vi "ATF-Pump-RT_DAQ.vi"(8 "error in":errorcluster, 11 "Data FIFO Ref":T1) -> (0 "error out":errorcluster)   [LabVIEW 2022 SP3]
uses:
  RT Controls/ATF-Pump-Data FIFO.ctl
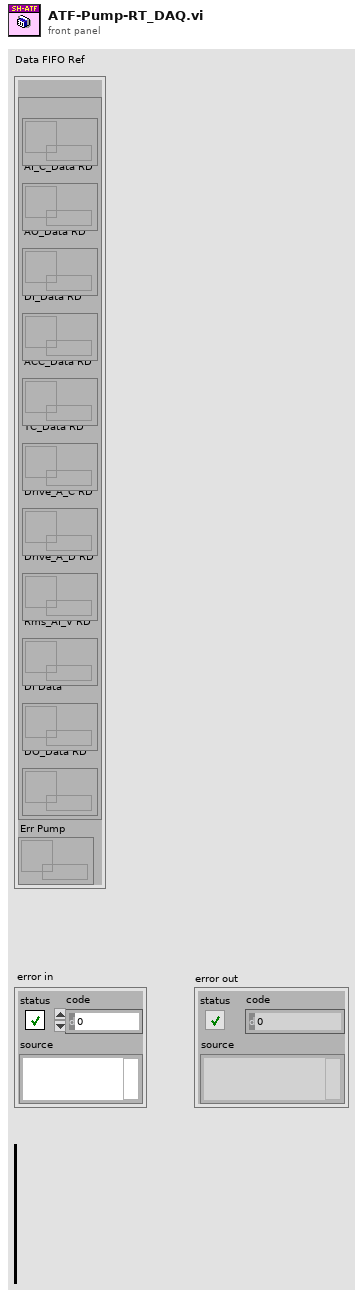
[diagram p1: front panel]
types:
  T1 = typedef "ATF-Pump-Data FIFO.ctl" = cluster{"RD":cluster{"AI_V_Data RD":refnum<queue>, "AI_C_Data RD":refnum<queue>, "AO_Data RD":refnum<queue>, "DI_Data RD":refnum<queue>, "ACC_Data RD":refnum<queue>, "TC_Data RD":refnum<queue>, "Drive_A_C RD":refnum<queue>, "Drive_A_D RD":refnum<queue>, "Rms_AI_V RD":refnum<queue>, "DI Data":refnum<queue>, "DO_Data RD":refnum<queue>}, "Err Pump":refnum<queue>}
  T2 = cluster{"Config":cluster{"AO config":cluster{"Channel_Name":string, "Channel_Number":string, "Default_Value":dbl, "Units":string}[], "AI config":cluster{"Channel_Name":string, "Channel_Number":string, "Pre_Scale_min":dbl, "Pre_Scale_max":dbl, "Sensor_min":dbl, "Sensor_max":dbl, "Units":string}[], "DI config":cluster{"Channel_Name":string, "Channel_Number":string, "Default_Value":bool, "DI invert?":bool}[], "DO config":cluster{"Channel_Name":string, "Channel_Number":string, "Default_Value":bool, "DO invert?":bool}[], "TC config":cluster{"Channel_Name":string, "Channel_Number":string, "Pre_Scale_min":dbl, "Pre_Scale_max":dbl, "units":i32, " type":i32}[], "ACC config":cluster{"Channel_Name":string, "Channel_Number":string, "Pre_Scale_min":dbl, "Pre_Scale_max":dbl, "Terminal configuration":i32, "Sensitivity":dbl, "Sensitivity units":i32}[], "SG config":cluster{"Channel_Name":string, "Channel_Number":string, "Pre_Scale_min":dbl, "Pre_Scale_max":dbl}[], "Strain Gauge Settings":cluster{"poisson ratio":dbl, "nominal gage resistance":dbl, "gage factor":dbl}, "Bridge Settings":cluster{"voltage excitation value":dbl, "voltage excitation source":i32, "initial bridge voltage":dbl, "lead wire resistance":dbl, "strain configuration":i32}, "Sample Rate":cluster{"AI Sample Rate":dbl[], "AO Sample Rate":dbl[], "DI Sample Rate":dbl[], "TC Sample Rate":dbl[], "DO Sample Rate":dbl[], "SG Sample Rate":dbl[], "ACC Sample Rate":dbl[]}}, "FIFO Ref":T1, "AI_Task":refnum<k21>, "AO_Task":refnum<k21>, "DI_Task":refnum<k21>, "DO_Task":refnum<k21>, "ACC_Task":refnum<k21>, "TC_Task":refnum<k21>, "AI_V_Task":refnum<k21>}
  T3 = enum16{"Initialize", "Create Task", "Start", "Acquire", "Stop", "Exit"}
  T4 = cluster{"Start DAQ":bool, "Stop DAQ":bool, "RT Stop":bool, "RT Exit":bool, "Start Seq":bool}
  T5 = cluster{"AO config":cluster{"Channel_Name":string, "Channel_Number":string, "Default_Value":dbl, "Units":string}[], "AI config":cluster{"Channel_Name":string, "Channel_Number":string, "Pre_Scale_min":dbl, "Pre_Scale_max":dbl, "Sensor_min":dbl, "Sensor_max":dbl, "Units":string}[], "DI config":cluster{"Channel_Name":string, "Channel_Number":string, "Default_Value":bool, "DI invert?":bool}[], "DO config":cluster{"Channel_Name":string, "Channel_Number":string, "Default_Value":bool, "DO invert?":bool}[], "TC config":cluster{"Channel_Name":string, "Channel_Number":string, "Pre_Scale_min":dbl, "Pre_Scale_max":dbl, "units":i32, "thermocouple type":i32}[], "ACC config":cluster{"Channel_Name":string, "Channel_Number":string, "Pre_Scale_min":dbl, "Pre_Scale_max":dbl, "Terminal configuration":i32, "Sensitivity":dbl, "Sensitivity units":i32}[], "SG config":cluster{"Channel_Name":string, "Channel_Number":string, "Pre_Scale_min":dbl, "Pre_Scale_max":dbl}[], "Strain Gauge Settings":cluster{"poisson ratio":dbl, "nominal gage resistance":dbl, "gage factor":dbl}, "Bridge Settings":cluster{"voltage excitation value":dbl, "voltage excitation source":i32, "initial bridge voltage":dbl, "lead wire resistance":dbl, "strain configuration":i32}, "Sample Rate":cluster{"AI Sample Rate":dbl[], "AO Sample Rate":dbl[], "DI Sample Rate":dbl[], "TC Sample Rate":dbl[], "DO Sample Rate":dbl[], "SG Sample Rate":dbl[], "ACC Sample Rate":dbl[]}}
  T6 = cluster{"Channel_Name":string, "Channel_Number":string, "Pre_Scale_min":dbl, "Pre_Scale_max":dbl, "Sensor_min":dbl, "Sensor_max":dbl, "Units":string}[]
  T7 = cluster{"Channel_Name":string, "Channel_Number":string, "Default_Value":dbl, "Units":string}[]
  T8 = cluster{"Channel_Name":string, "Channel_Number":string, "Default_Value":bool, "DI invert?":bool}[]
  T9 = cluster{"Channel_Name":string, "Channel_Number":string, "Default_Value":bool, "DO invert?":bool}[]
  T10 = cluster{"Channel_Name":string, "Channel_Number":string, "Pre_Scale_min":dbl, "Pre_Scale_max":dbl, "Terminal configuration":i32, "Sensitivity":dbl, "Sensitivity units":i32}[]
  T11 = cluster{"Channel_Name":string, "Channel_Number":string, "Pre_Scale_min":dbl, "Pre_Scale_max":dbl, "units":i32, " type":i32}[]
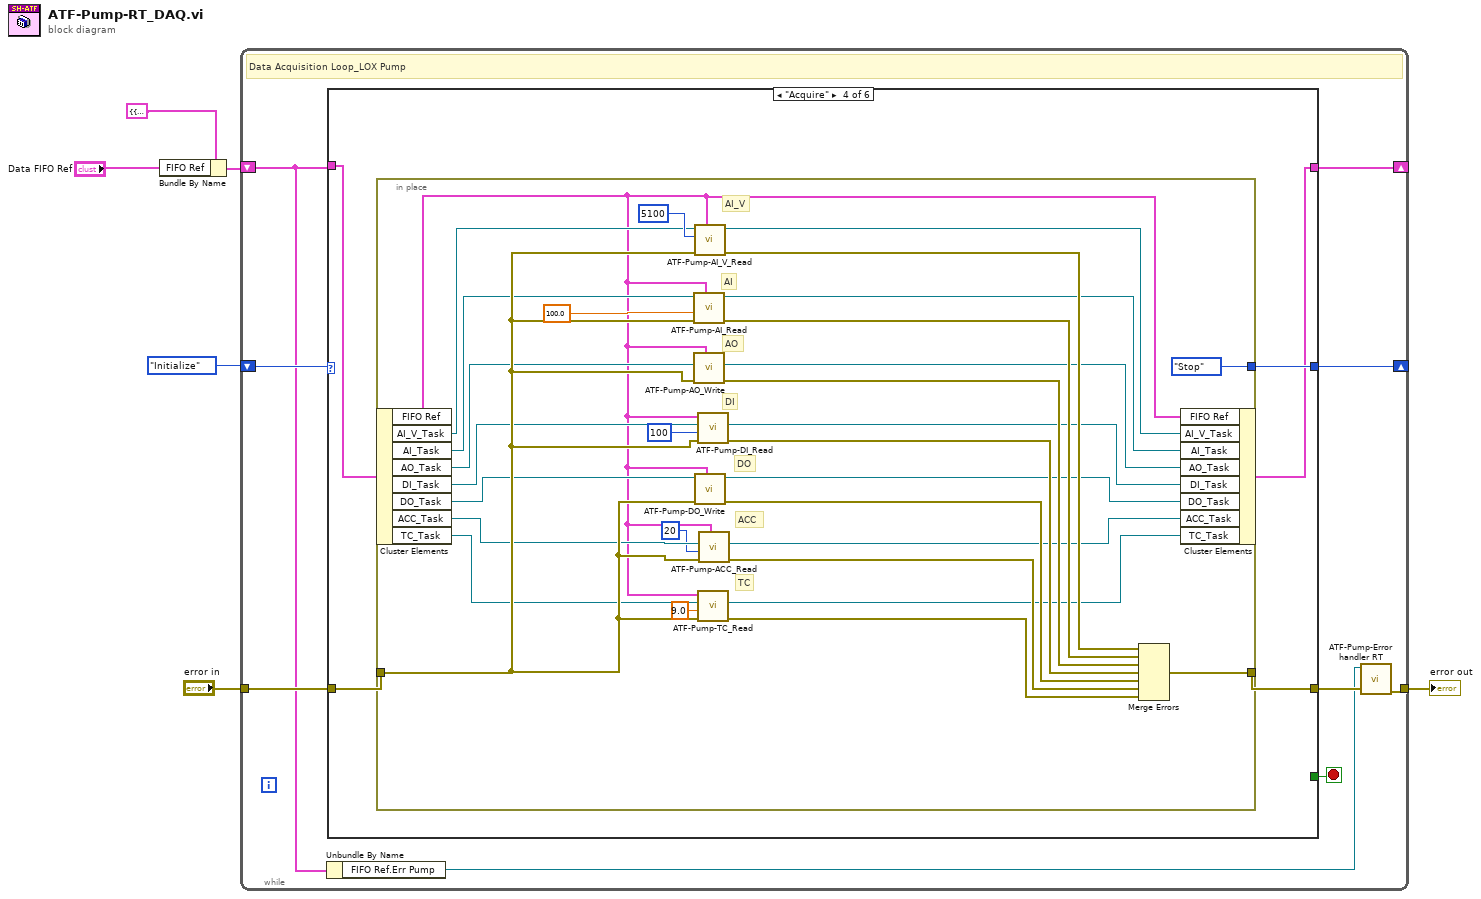
[diagram p0: block diagram]
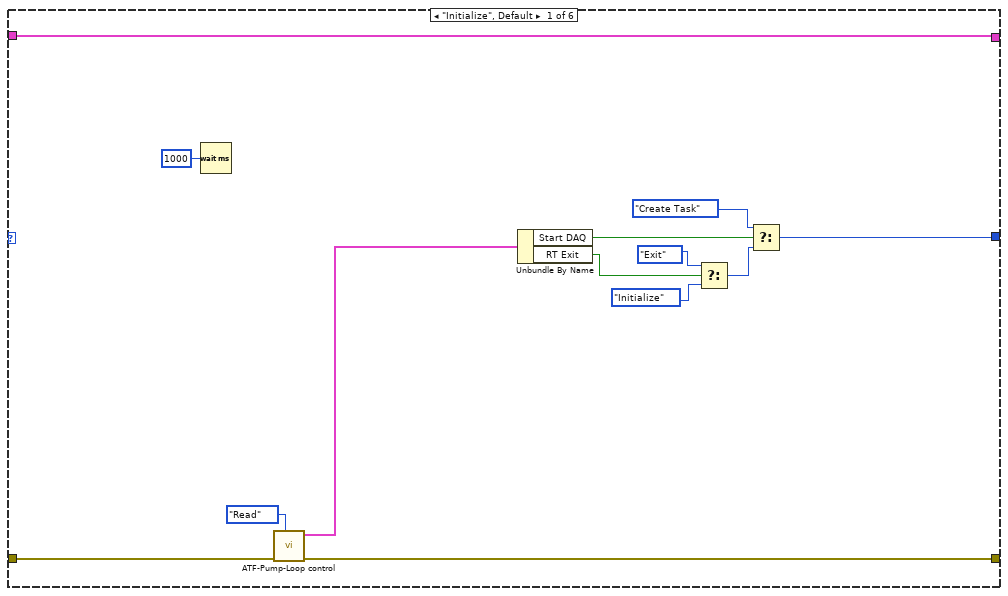
[diagram p2: hidden frame]
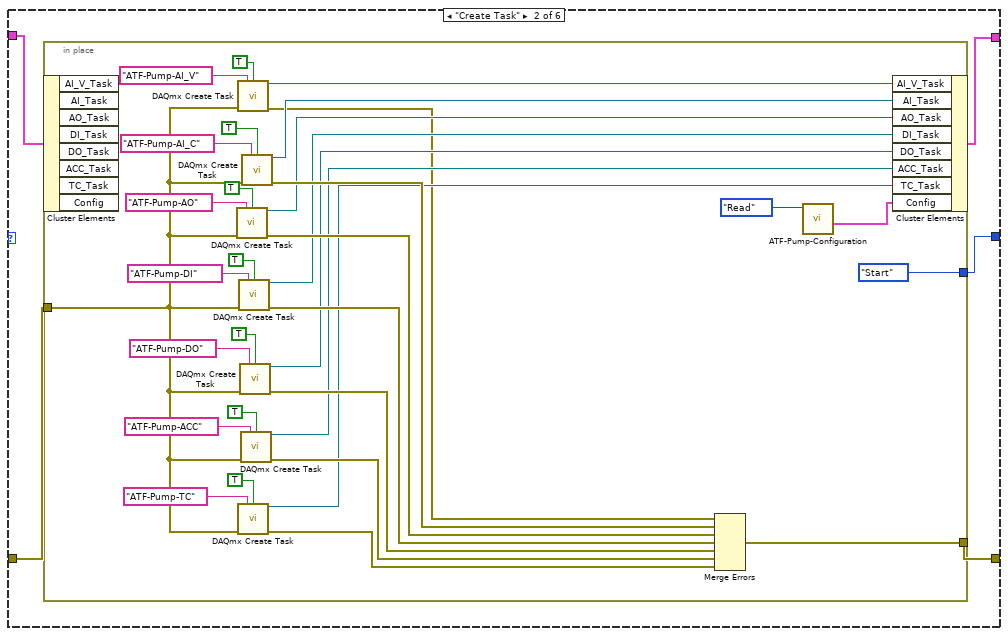
[diagram p3: hidden frame]
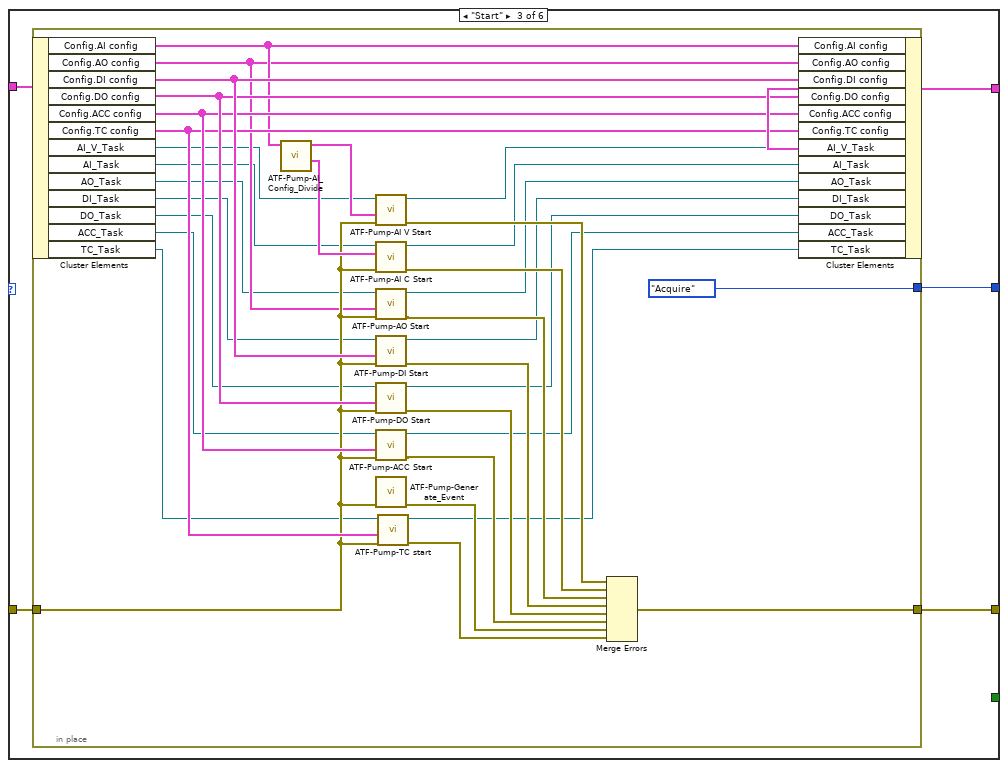
[diagram p4: hidden frame]
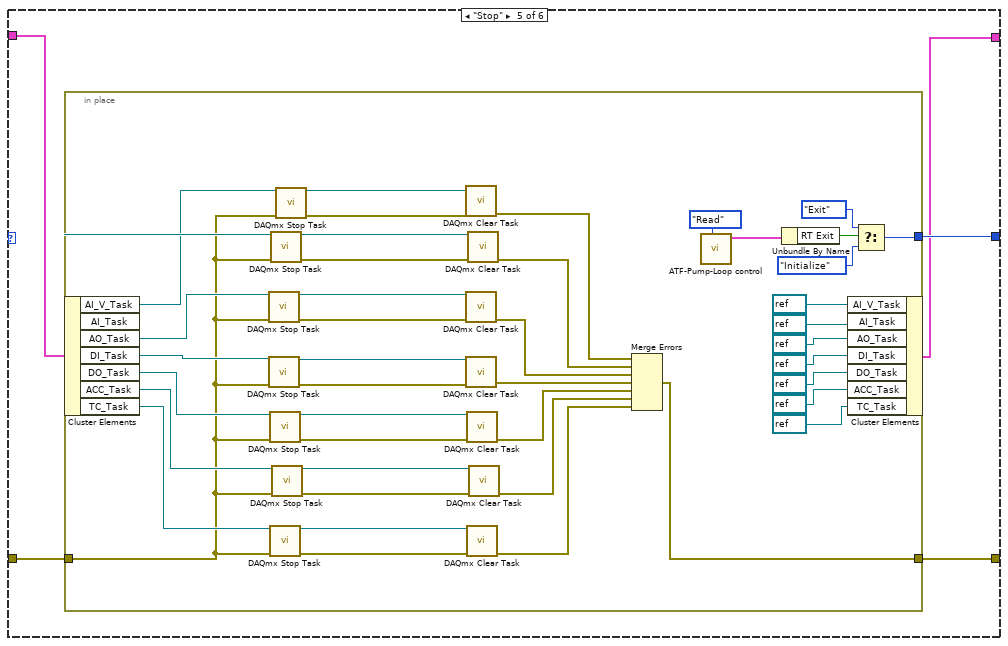
[diagram p5: hidden frame]
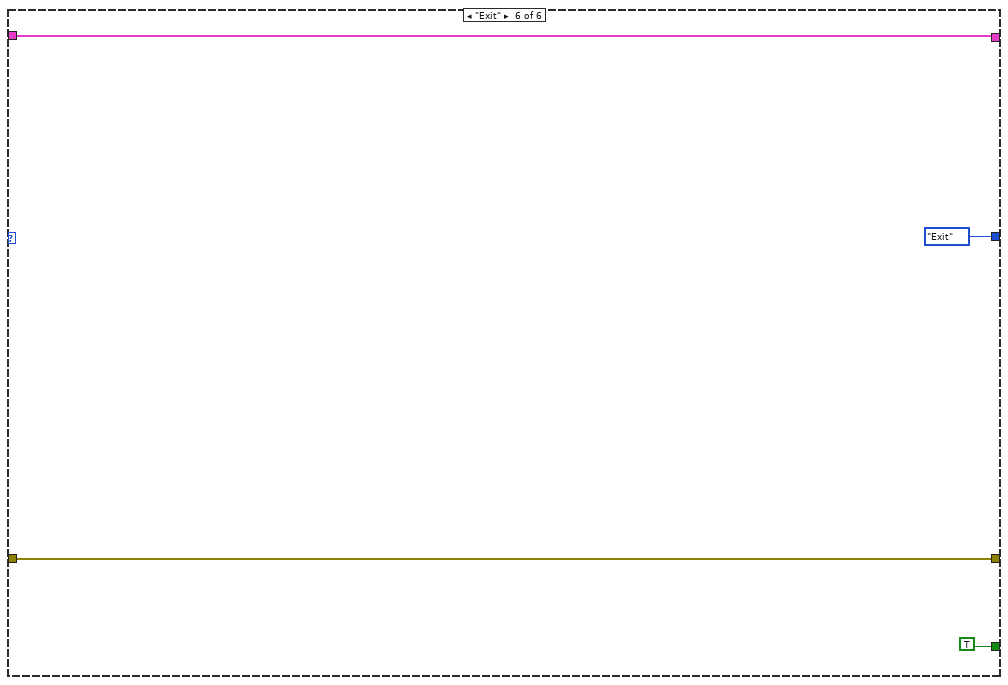
[diagram p6: hidden frame]
diagram:
  n1 = Bundle By Name(cluster=T2 {"Config"={"AO config"=[], "AI config"=[], "DI config"=[], "DO config"=[], "TC config"=[], "ACC config"=[], "SG config"=[], "Strain Gauge Settings"={"poisson ratio"=0.0, "nominal gage resistance"=0.0, "gage factor"=0.0}, "Bridge Settings"={"voltage excitation value"=0.0, "voltage excitation source"=0, "initial bridge voltage"=0.0, "lead wire resistance"=0.0, "strain configuration"=0}, "Sample Rate"={"AI Sample Rate"=[], "AO Sample Rate"=[], "DI Sample Rate"=[], "TC Sample Rate"=[], "DO Sample Rate"=[], "SG Sample Rate"=[], "ACC Sample Rate"=[]}}, "FIFO Ref"={"RD"={"AI_V_Data RD"=refnum, "AI_C_Data RD"=refnum, "AO_Data RD"=refnum, "DI_Data RD"=refnum, "ACC_Data RD"=refnum, "TC_Data RD"=refnum, "Drive_A_C RD"=refnum, "Drive_A_D RD"=refnum, "Rms_AI_V RD"=refnum, "DI Data"=refnum, "DO_Data RD"=refnum}, "Err Pump"=refnum}, "AI_Task"="", "AO_Task"="", "DI_Task"="", "DO_Task"="", "ACC_Task"="", "TC_Task"="", "AI_V_Task"=""}, "FIFO Ref"="Data FIFO Ref") -> (w3:T2)
  n2 = while {
    shift-right: [w13] -> _
    shift-left: T3."Initialize" -> [w15]
    tunnel: "error in" -> [w14]
    tunnel: [w9] -> w5
    shift-right: [w12] -> _
    shift-left: w3 -> [w8]
    stop <- w11 stop-if-true
    # "Data Acquisition Loop_LOX Pump"
    n3 = Unbundle By Name(w8) -> ("FIFO Ref.Err Pump"=w7:refnum<queue>)
    n4 = case shown="\"Acquire\"" w15 {
      tunnel: w14 -> [w18 w33 w70 w108 w142 w188]
      tunnel: [w17 w32 w69 w107 w143 w188] -> w10
      tunnel: [w27 w31 w71 w109 w144 T3."Exit"] -> w13
      tunnel: w8 -> [w19 w30 w68 w105 w141 w189]
      tunnel: [w19 w29 w67 w106 w140 w189] -> w12
      tunnel: [_ _ _ _ _ TRUE] -> w11
      frame "Initialize", Default {
        n5 = Wait (ms)(milliseconds to wait=u32 1000) -> ()  [unwired: 1 out]
        n6 = call "ATF-Pump-Loop control.vi"("Action"=enum16{"Init", "Write", "Read"}."Read", "error in (no error)"=w18) -> ("error Out"=w17:errorcluster, "Loop Control out"=w23:T4)  [unwired: 8 in]
        n7 = Unbundle By Name(w23) -> ("Start DAQ"=w22:bool, "RT Exit"=w21:bool)
        n8 = Select(t=T3."Exit", s=w21, f=T3."Initialize") -> (s? t:f=w24:T3)
        n9 = Select(t=T3."Create Task", s=w22, f=w24) -> (s? t:f=w27:T3)
      }
      frame "Create Task" {
        n10 = in-place "In Place Element Structure" {
          in-place-border: w33 -> [w35]
          in-place-border: [w55] -> w32
          in-place-border: [T3."Start"] -> w31
          n11 = in-place-cluster #1(w30) -> ()  [unwired: 8 out]
          n12 = call <vilib>:"DAQmx Create Task.vi"("new task name"="ATF-Pump-AO", "auto cleanup"=TRUE, "error in"=w35) -> ("task out"=w53:refnum<k21>, "error out"=w60:errorcluster)  [unwired: 11 in]
          n13 = call <vilib>:"DAQmx Create Task.vi"("new task name"="ATF-Pump-AI_V", "auto cleanup"=TRUE, "error in"=w35) -> ("task out"=w46:refnum<k21>, "error out"=w36:errorcluster)  [unwired: 11 in]
          n14 = call <vilib>:"DAQmx Create Task.vi"("new task name"="ATF-Pump-TC", "auto cleanup"=TRUE, "error in"=w35) -> ("task out"=w49:refnum<k21>, "error out"=w56:errorcluster)  [unwired: 11 in]
          n15 = call <vilib>:"DAQmx Create Task.vi"("new task name"="ATF-Pump-DI", "auto cleanup"=TRUE, "error in"=w35) -> ("task out"=w52:refnum<k21>, "error out"=w59:errorcluster)  [unwired: 11 in]
          n16 = call <vilib>:"DAQmx Create Task.vi"("new task name"="ATF-Pump-DO", "auto cleanup"=TRUE, "error in"=w35) -> ("task out"=w51:refnum<k21>, "error out"=w58:errorcluster)  [unwired: 11 in]
          n17 = call <vilib>:"DAQmx Create Task.vi"("new task name"="ATF-Pump-ACC", "auto cleanup"=TRUE, "error in"=w35) -> ("task out"=w50:refnum<k21>, "error out"=w57:errorcluster)  [unwired: 11 in]
          n18 = call <vilib>:"DAQmx Create Task.vi"("new task name"="ATF-Pump-AI_C", "auto cleanup"=TRUE, "error in"=w35) -> ("task out"=w54:refnum<k21>, "error out"=w66:errorcluster)  [unwired: 11 in]
          n19 = Merge Errors(w36, w66, w60, w59, w58, w57, w56) -> (w55:errorcluster)
          n20 = call "ATF-Pump-Configuration.vi"("Enum"=enum16{"Write", "Read"}."Read") -> ("Config out"=w34:T5)  [unwired: 10 in]
          n21 = in-place-cluster #1("AI_V_Task"=w46, "AI_Task"=w54, "AO_Task"=w53, "DI_Task"=w52, "DO_Task"=w51, "ACC_Task"=w50, "TC_Task"=w49, "Config"=w34) -> (w29:T2)
        }
      }
      frame "Start" {
        n22 = in-place "In Place Element Structure" {
          in-place-border: [T3."Acquire"] -> w71
          in-place-border: w70 -> [w92]
          in-place-border: [w87] -> w69
          n23 = in-place-cluster #2(w68) -> ("Config.AI config"=w99:T6, "Config.AO config"=w86:T7, "Config.DI config"=w103:T8, "Config.DO config"=w102:T9, "Config.ACC config"=w101:T10, "Config.TC config"=w100:T11, "AI_V_Task"=w85:refnum<k21>, "AI_Task"=w83:refnum<k21>, "AO_Task"=w81:refnum<k21>, "DI_Task"=w80:refnum<k21>, "DO_Task"=w79:refnum<k21>, "ACC_Task"=w78:refnum<k21>, "TC_Task"=w77:refnum<k21>)
          n24 = call "ATF-Pump-AI_Config_Divide.vi"("AI config"=w99) -> ("AI C"=w97:T6, "AI V"=w98:T6)  [unwired: 9 in]
          n25 = call "ATF-Pump-AI V Start.vi"("error in"=w92, "AI V"=w98, "Refnum in"=w85) -> ("error out"=w96:errorcluster, "Refnum out"=w84:refnum<k21>)  [unwired: 7 in]
          n26 = call "ATF-Pump-AI C Start.vi"("error in"=w92, "AI C"=w97, "Refnum in"=w83) -> ("error out"=w95:errorcluster, "Refnum out"=w82:refnum<k21>)  [unwired: 7 in]
          n27 = call "ATF-Pump-AO Start.vi"("error in"=w92, "AO config"=w86, "Refnum in"=w81) -> ("error out"=w94:errorcluster, "Refnum out"=w76:refnum<k21>)  [unwired: 7 in]
          n28 = call "ATF-Pump-DI Start.vi"("error in"=w92, "DI config"=w103, "Refnum in"=w80) -> ("error out"=w93:errorcluster, "Refnum out"=w75:refnum<k21>)  [unwired: 7 in]
          n29 = call "ATF-Pump-DO Start.vi"("error in"=w92, "DO config"=w102, "Refnum in"=w79) -> ("error out"=w91:errorcluster, "Refnum out"=w74:refnum<k21>)  [unwired: 7 in]
          n30 = call "ATF-Pump-ACC Start.vi"("error in"=w92, "ACC config"=w101, "Refnum in"=w78) -> ("error out"=w90:errorcluster, "Refnum out"=w73:refnum<k21>)  [unwired: 7 in]
          n31 = call "ATF-Pump-Generate_Event.vi"("error in"=w92) -> ("error out"=w89:errorcluster)  [unwired: 10 in]
          n32 = call "ATF-Pump-TC start.vi"("error in"=w92, "TC config"=w100, "Refnum in"=w77) -> ("error out"=w88:errorcluster, "Refnum out"=w72:refnum<k21>)  [unwired: 7 in]
          n33 = Merge Errors(w96, w95, w94, w93, w91, w90, w89, w88) -> (w87:errorcluster)
          n34 = in-place-cluster #2("Config.AI config"=w99, "Config.AO config"=w86, "Config.DI config"=w103, "Config.DO config"=w102, "Config.ACC config"=w101, "Config.TC config"=w100, "AI_V_Task"=w84, "AI_Task"=w82, "AO_Task"=w76, "DI_Task"=w75, "DO_Task"=w74, "ACC_Task"=w73, "TC_Task"=w72) -> (w67:T2)
        }
      }
      frame "Acquire" {
        n35 = in-place "In Place Element Structure" {
          in-place-border: [T3."Stop"] -> w109
          in-place-border: w108 -> [w130]
          in-place-border: [w138] -> w107
          # "ACC"
          # "AO"
          # "AI_V"
          # "TC"
          # "DO"
          # "DI"
          # "AI"
          n36 = in-place-cluster #3(w105) -> ("FIFO Ref"=w110:T1, "AI_V_Task"=w114:refnum<k21>, "AI_Task"=w128:refnum<k21>, "AO_Task"=w127:refnum<k21>, "DI_Task"=w126:refnum<k21>, "DO_Task"=w125:refnum<k21>, "ACC_Task"=w124:refnum<k21>, "TC_Task"=w123:refnum<k21>)
          n37 = call "ATF-Pump-AI_Read.vi"("Data FIFO Ref"=w110, "error in (no error)"=w130, "Numeric"=100.0, "AI_Task"=w128) -> ("error out"=w136:errorcluster, "task out"=w121:refnum<k21>)  [unwired: 4 in]
          n38 = call "ATF-Pump-AO_Write.vi"("Data FIFO Ref"=w110, "error in (no error)"=w130, "AO_Task"=w127) -> ("error out"=w135:errorcluster, "task out"=w120:refnum<k21>)  [unwired: 7 in]
          n39 = call "ATF-Pump-AI_V_Read.vi"("Data FIFO Ref"=w110, "error in"=w130, "number of samples per channel"=5100, "AI_V_Task"=w114) -> ("error out"=w137:errorcluster, "AI_V_Task"=w122:refnum<k21>)  [unwired: 6 in]
          n40 = call "ATF-Pump-DO_Write.vi"("Data FIFO Ref"=w110, "error in (no error)"=w130, "Refnum in"=w125) -> ("error out"=w133:errorcluster, "Refnum out"=w118:refnum<k21>)  [unwired: 7 in]
          n41 = call "ATF-Pump-DI_Read.vi"("error in (no error)"=w130, "number of samples per channel"=100, "DI_Task"=w126, "Data FIFO Ref"=w110) -> ("error out"=w134:errorcluster, "task out"=w119:refnum<k21>)  [unwired: 6 in]
          n42 = call "ATF-Pump-TC_Read.vi"("error in (no error)"=w130, "Numeric"=9.0, "TC_Task"=w123, "Data FIFO Ref"=w110) -> ("error out"=w131:errorcluster, "task out"=w116:refnum<k21>)  [unwired: 6 in]
          n43 = call "ATF-Pump-ACC_Read.vi"("Data FIFO Ref"=w110, "error in (no error)"=w130, "number of samples per channel"=20, "ACC_Task"=w124) -> ("error out"=w132:errorcluster, "task out"=w117:refnum<k21>)  [unwired: 6 in]
          n44 = Merge Errors(w137, w136, w135, w134, w133, w132, w131) -> (w138:errorcluster)
          n45 = in-place-cluster #3("FIFO Ref"=w110, "AI_V_Task"=w122, "AI_Task"=w121, "AO_Task"=w120, "DI_Task"=w119, "DO_Task"=w118, "ACC_Task"=w117, "TC_Task"=w116) -> (w106:T2)
        }
      }
      frame "Stop" {
        n46 = in-place "In Place Element Structure" {
          in-place-border: [w184] -> w144
          in-place-border: [w178] -> w143
          in-place-border: w142 -> [w159]
          n47 = in-place-cluster #4(w141) -> ("AI_V_Task"=w161:refnum<k21>, "AI_Task"=w170:refnum<k21>, "AO_Task"=w169:refnum<k21>, "DI_Task"=w172:refnum<k21>, "DO_Task"=w171:refnum<k21>, "ACC_Task"=w168:refnum<k21>, "TC_Task"=w167:refnum<k21>)
          n48 = call <vilib>:"DAQmx Stop Task.vi"("task/channels in"=w169, "error in"=w159) -> ("task out"=w166:refnum<k21>, "error out"=w183:errorcluster)  [unwired: 12 in]
          n49 = call <vilib>:"DAQmx Stop Task.vi"("task/channels in"=w172, "error in"=w159) -> ("task out"=w165:refnum<k21>, "error out"=w182:errorcluster)  [unwired: 12 in]
          n50 = call <vilib>:"DAQmx Stop Task.vi"("task/channels in"=w171, "error in"=w159) -> ("task out"=w164:refnum<k21>, "error out"=w181:errorcluster)  [unwired: 12 in]
          n51 = call <vilib>:"DAQmx Stop Task.vi"("task/channels in"=w167, "error in"=w159) -> ("task out"=w162:refnum<k21>, "error out"=w179:errorcluster)  [unwired: 12 in]
          n52 = call <vilib>:"DAQmx Stop Task.vi"("task/channels in"=w170, "error in"=w159) -> ("task out"=w147:refnum<k21>, "error out"=w146:errorcluster)  [unwired: 12 in]
          n53 = call <vilib>:"DAQmx Stop Task.vi"("task/channels in"=w168, "error in"=w159) -> ("task out"=w163:refnum<k21>, "error out"=w180:errorcluster)  [unwired: 12 in]
          n54 = call <vilib>:"DAQmx Stop Task.vi"("task/channels in"=w161, "error in"=w159) -> ("task out"=w160:refnum<k21>, "error out"=w158:errorcluster)  [unwired: 12 in]
          n55 = call <vilib>:"DAQmx Clear Task.vi"("task in"=w160, "error in"=w158) -> ("error out"=w157:errorcluster)  [unwired: 13 in]
          n56 = call <vilib>:"DAQmx Clear Task.vi"("task in"=w166, "error in"=w183) -> ("error out"=w177:errorcluster)  [unwired: 13 in]
          n57 = call <vilib>:"DAQmx Clear Task.vi"("task in"=w165, "error in"=w182) -> ("error out"=w176:errorcluster)  [unwired: 13 in]
          n58 = call <vilib>:"DAQmx Clear Task.vi"("task in"=w164, "error in"=w181) -> ("error out"=w175:errorcluster)  [unwired: 13 in]
          n59 = call <vilib>:"DAQmx Clear Task.vi"("task in"=w162, "error in"=w179) -> ("error out"=w173:errorcluster)  [unwired: 13 in]
          n60 = call <vilib>:"DAQmx Clear Task.vi"("task in"=w147, "error in"=w146) -> ("error out"=w187:errorcluster)  [unwired: 13 in]
          n61 = call <vilib>:"DAQmx Clear Task.vi"("task in"=w163, "error in"=w180) -> ("error out"=w174:errorcluster)  [unwired: 13 in]
          n62 = Merge Errors(w157, w187, w177, w176, w175, w174, w173) -> (w178:errorcluster)
          n63 = call "ATF-Pump-Loop control.vi"("Action"=enum16{"Init", "Write", "Read"}."Read") -> ("Loop Control out"=w156:T4)  [unwired: 9 in, 1 out]
          n64 = Unbundle By Name(w156) -> ("RT Exit"=w155:bool)
          n65 = in-place-cluster #4("AI_V_Task"=refnum<k21> refnum, "AI_Task"=refnum<k21> refnum, "AO_Task"=refnum<k21> refnum, "DI_Task"=refnum<k21> refnum, "DO_Task"=refnum<k21> refnum, "ACC_Task"=refnum<k21> refnum, "TC_Task"=refnum<k21> refnum) -> (w140:T2)
          n66 = Select(t=T3."Exit", s=w155, f=T3."Initialize") -> (s? t:f=w184:T3)
        }
      }
      frame "Exit" {
      }
    }
    n67 = call "ATF-Pump-Error handler RT.vi"("error in"=w10, "Message Queue"=w7) -> ("error out"=w9:errorcluster)  [unwired: 8 in, 1 out]
  }
  "error out" <- w5
